vi "Insert bit in Byte.vi"(3 "Value":bool, 4 "Input (hex)":u8 format="0x%x", 5 "bit":u8) -> (1 "output (hex)":u32 format="0x%x")   [LabVIEW 2021]
panel:
  out "output":bool[](array[boolean])
  out "Input":bool[](array[boolean])
  # "7"
  # "6"
  # "5"
  # "4"
  # "3"
  # "2"
  # "1"
  # "0"
  # "7"
  # "6"
  # "5"
  # "4"
  # "3"
  # "2"
  # "1"
  # "0"
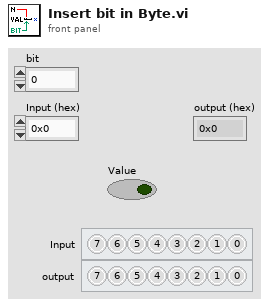
[diagram p1: front panel]
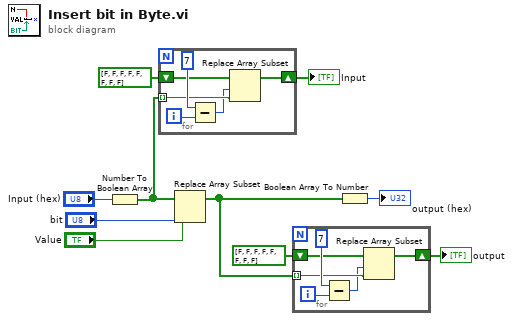
[diagram p0: block diagram]
diagram:
  n1 = Number To Boolean Array(number="Input (hex)") -> (Boolean array=w6:bool[])
  n2 = for {
    tunnel: w6 -> [w12] mode=indexing
    shift-right: [w13] -> w1
    shift-left: bool[] [FALSE, FALSE, FALSE, FALSE, FALSE, FALSE, FALSE, FALSE] ("array") -> [w14]
    i -> [w15]
    n3 = Subtract(x=7 ("y"), y=w15) -> (x-y=w11:i32)
    n4 = Replace Array Subset(array=w14, new element=w12, index=w11) -> (w13:bool[])
  }
  "Input" <- w1
  n5 = Replace Array Subset(array=w6, new element="Value", index="bit") -> (w3:bool[])
  n6 = for {
    tunnel: w3 -> [w18] mode=indexing
    shift-right: [w19] -> w2
    shift-left: bool[] [FALSE, FALSE, FALSE, FALSE, FALSE, FALSE, FALSE, FALSE] ("array") -> [w20]
    i -> [w21]
    n7 = Subtract(x=7 ("y"), y=w21) -> (x-y=w17:i32)
    n8 = Replace Array Subset(array=w20, new element=w18, index=w17) -> (w19:bool[])
  }
  "output" <- w2
  n9 = Boolean Array To Number(Boolean array=w3) -> (number=→"output (hex)":u32)
